vi "TEST-JSONtext-.vi"() -> ()   [LabVIEW 2019]
uses:
  3bf779cc-927d-47fd-9a8c-dc02e83297dd.vi
  <vilib>/numeric/Random Number (Range) U64.vi
  JSON-RPC/JSON-RPC.lvclass
  <vilib>/numeric/Random Number (Range) DBL.vi
  <vilib>/numeric/Random Number (Range) I64.vi
  db3575da-bffe-4b9a-a9e7-21096011e894.vi
  6d6a3817-36ec-47d6-89d3-dba7abc61dde.vi
  78cd6d8b-e620-455a-a055-8660cd06f8d0.vi
  2869ab1d-aaab-4e4d-b56e-11c366621307.vi
  740e50dd-5288-45d9-afe7-7378590220d4.vi
  7927d975-b5b9-47a3-92b0-890a8d5b504b.vi
  cbe2aa51-b106-4e40-bfc3-1c3b870f7b4b.vi
  <vilib>/ErrorRing/Error Ring.xnode
panel:
  out "spreadsheet string":string
  out "XY Graph":cluster{dbl[], dbl[]}[](graph)
  out "total":dbl format="%#_6p"
  in  "Max Response Size":i32=10000
  out "4. parse response":dbl format="%#_6p"
  out "3. create response":dbl format="%#_6p"
  out "2. parse request":dbl format="%#_6p"
  out "1. create request":dbl format="%#_6p"
  in  "method 2":string="pickFruit"
  in  "Params Type":enum16{"Array", "Cluster", "Single"}(ring)=enum."Cluster"
  in  "Num Type":enum16{"U64", "I64", "DBL"}(ring)=enum."I64"
  in  "params 2":T1={"param1"=0, "param2"=10, "param3"=10, "param2 2"=10}
  out "params":string
  out "<JSON> REQ":string
  out "error out":errorcluster
  out "id":string
  out "method":string
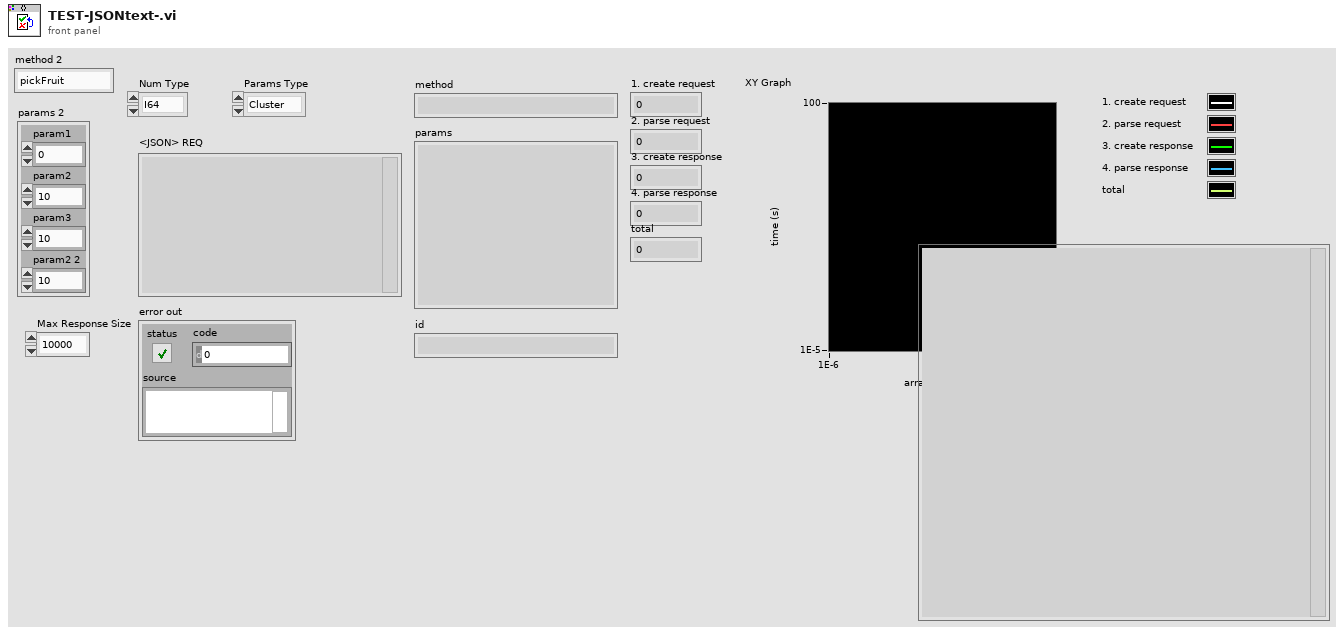
[diagram p1: front panel]
types:
  T1 = cluster{"param1":i32, "param2":i32, "param3":i32, "param2 2":i32}
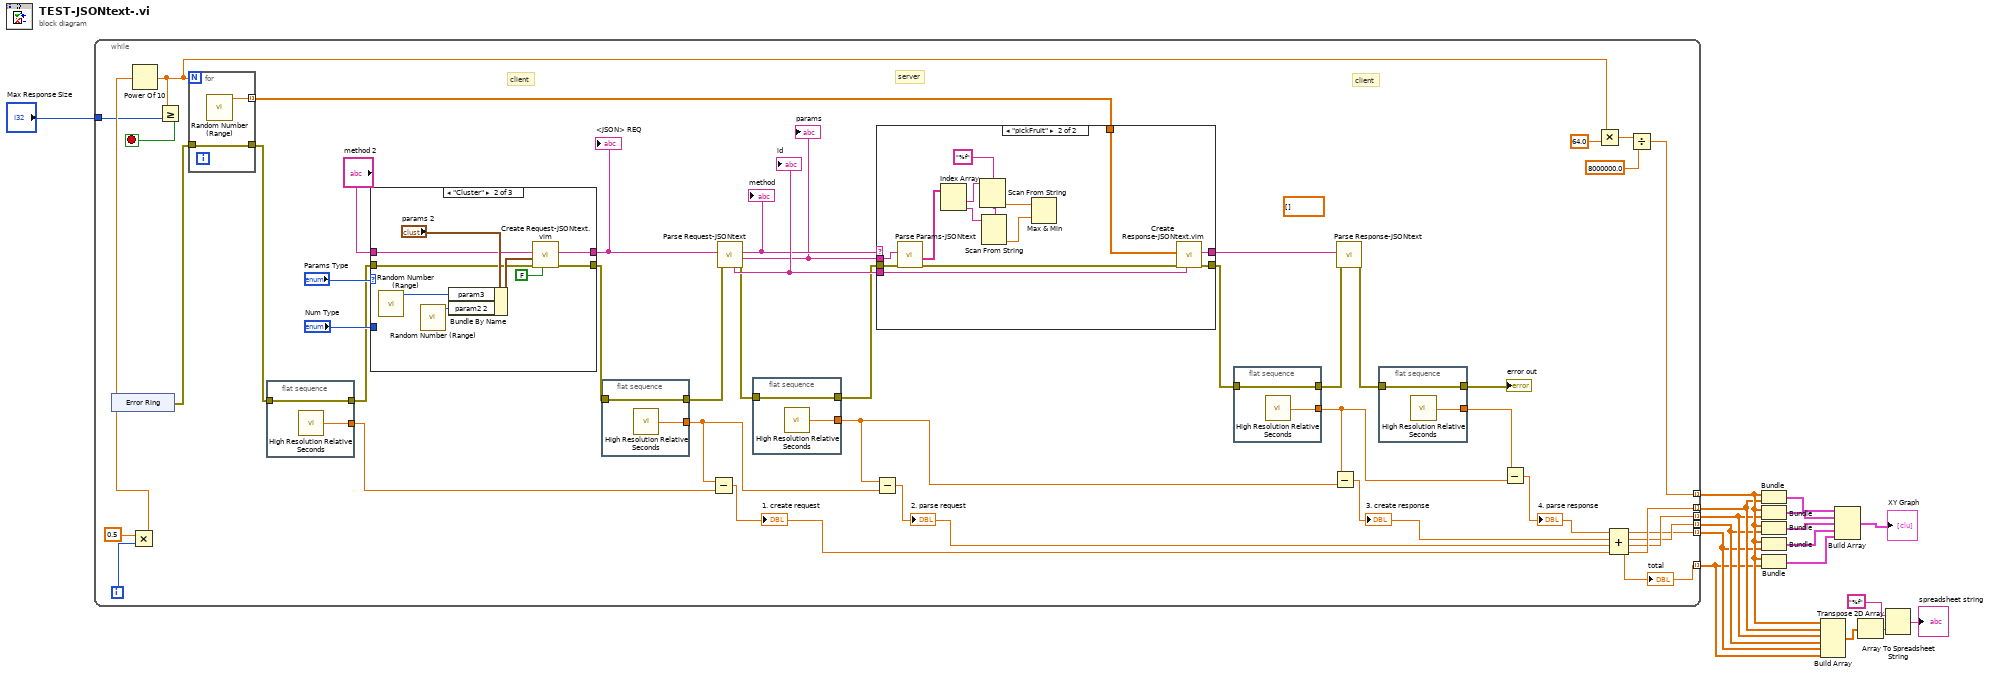
[diagram p0: block diagram]
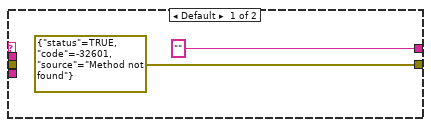
[diagram p2: hidden frame]
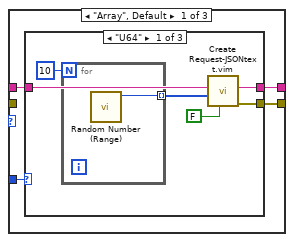
[diagram p3: hidden frame]
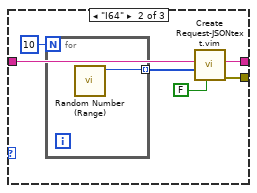
[diagram p4: hidden frame]
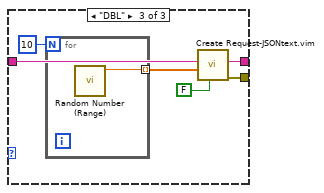
[diagram p5: hidden frame]
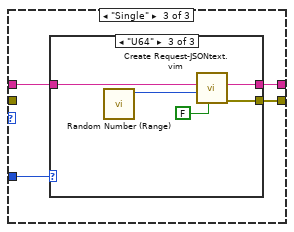
[diagram p6: hidden frame]
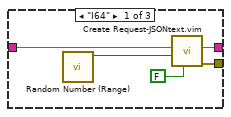
[diagram p7: hidden frame]
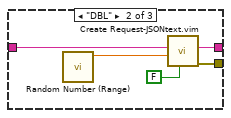
[diagram p8: hidden frame]
diagram:
  n1 = while {
    tunnel: [w32] -> w5 mode=indexing
    tunnel: [w31] -> w4 mode=indexing
    tunnel: [w30] -> w3 mode=indexing
    tunnel: [w29] -> w2 mode=indexing
    tunnel: [w28] -> w1 mode=indexing
    tunnel: [w25] -> w6 mode=indexing
    tunnel: "Max Response Size" -> [w19]
    i -> [w22]
    stop <- w18 stop-if-true
    (unwired) dbl[] []
    # "client"
    # "server"
    # "client"
    n2 = xnode "Error Ring"() -> ("error out"=w39:errorcluster)
    n3 = Multiply(x=0.5, y=w22) -> (x*y=w21:dbl)
    n4 = Power Of 10(x=w21) -> (10^x=w20:dbl)
    n5 = Greater Or Equal?(x=w20, y=w19) -> (x >= y?=w18:bool)
    n6 = for {
      N: w20 -> [_]
      tunnel: [w138] -> w33 mode=indexing
      tunnel: [w137] -> w40
      tunnel: w39 -> [w137]
      n7 = call-poly <vilib>:"Random Number (Range).vi"() -> ("number"=w138:dbl)  [unwired: 11 in]
    }
    n8 = flat-sequence {
      tunnel: w40 -> [w67]
      tunnel: [w67] -> w41
      tunnel: [w66] -> w38
      frame #0 {
        n9 = call <vilib>:"High Resolution Relative Seconds.vi"() -> ("relative seconds"=w66:dbl)
      }
    }
    n10 = case shown="\"Cluster\"" "Params Type" {
      tunnel: "Num Type" -> [w83 _ w120]
      tunnel: "method 2" -> [w84 w111 w119]
      tunnel: [w85 w110 w118] -> w49
      tunnel: [w86 w109 w117] -> w55
      tunnel: w41 -> [_ w108 _]
      frame "Array", Default {
        n11 = case shown="\"U64\"" w83 {
          tunnel: [w89 w95 w103] -> w86
          tunnel: [w90 w94 w102] -> w85
          tunnel: w84 -> [w87 w96 w101]
          frame "U64" {
            n12 = for {
              N: 10 -> [_]
              tunnel: [w93] -> w88 mode=indexing
              n13 = call-poly <vilib>:"Random Number (Range).vi"() -> ("number"=w93:u64)  [unwired: 11 in]
            }
            n14 = call "Create Request-JSONtext.vim"("notification?"=FALSE, "params"=w88, "method"=w87) -> ("error out"=w90:errorcluster, "{JSON}"=w89:string)  [unwired: 6 in, 1 out]
          }
          frame "I64" {
            n15 = for {
              N: 10 -> [_]
              tunnel: [w100] -> w97 mode=indexing
              n16 = call-poly <vilib>:"Random Number (Range).vi"() -> ("number"=w100:i64)  [unwired: 11 in]
            }
            n17 = call "Create Request-JSONtext.vim"("notification?"=FALSE, "params"=w97, "method"=w96) -> ("error out"=w94:errorcluster, "{JSON}"=w95:string)  [unwired: 6 in, 1 out]
          }
          frame "DBL" {
            n18 = for {
              N: 10 -> [_]
              tunnel: [w107] -> w104 mode=indexing
              n19 = call-poly <vilib>:"Random Number (Range).vi"() -> ("number"=w107:dbl)  [unwired: 11 in]
            }
            n20 = call "Create Request-JSONtext.vim"("notification?"=FALSE, "params"=w104, "method"=w101) -> ("error out"=w102:errorcluster, "{JSON}"=w103:string)  [unwired: 6 in, 1 out]
          }
        }
      }
      frame "Cluster" {
        n21 = call-poly <vilib>:"Random Number (Range).vi"() -> ("number"=w114:u64)  [unwired: 11 in]
        n22 = call-poly <vilib>:"Random Number (Range).vi"() -> ("number"=w115:u64)  [unwired: 11 in]
        n23 = Bundle By Name(cluster="params 2", "param3"=w114, "param2 2"=w115) -> (w112:T1)
        n24 = call "Create Request-JSONtext.vim"("notification?"=FALSE, "error in (no error)"=w108, "params"=w112, "method"=w111) -> ("error out"=w110:errorcluster, "{JSON}"=w109:string)  [unwired: 5 in, 1 out]
      }
      frame "Single" {
        n25 = case shown="\"U64\"" w120 {
          tunnel: w119 -> [w124 w129 w133]
          tunnel: [w123 w126 w131] -> w118
          tunnel: [w122 w127 w132] -> w117
          frame "I64" {
            n26 = call-poly <vilib>:"Random Number (Range).vi"() -> ("number"=w121:i64)  [unwired: 11 in]
            n27 = call "Create Request-JSONtext.vim"("notification?"=FALSE, "params"=w121, "method"=w124) -> ("error out"=w123:errorcluster, "{JSON}"=w122:string)  [unwired: 6 in, 1 out]
          }
          frame "DBL" {
            n28 = call-poly <vilib>:"Random Number (Range).vi"() -> ("number"=w128:dbl)  [unwired: 11 in]
            n29 = call "Create Request-JSONtext.vim"("notification?"=FALSE, "params"=w128, "method"=w129) -> ("error out"=w126:errorcluster, "{JSON}"=w127:string)  [unwired: 6 in, 1 out]
          }
          frame "U64" {
            n30 = call-poly <vilib>:"Random Number (Range).vi"() -> ("number"=w134:u64)  [unwired: 11 in]
            n31 = call "Create Request-JSONtext.vim"("notification?"=FALSE, "params"=w134, "method"=w133) -> ("error out"=w131:errorcluster, "{JSON}"=w132:string)  [unwired: 6 in, 1 out]
          }
        }
      }
    }
    "<JSON> REQ" <- w55
    n32 = flat-sequence {
      tunnel: w49 -> [w65]
      tunnel: [w65] -> w48
      tunnel: [w64] -> w37
      frame #0 {
        n33 = call <vilib>:"High Resolution Relative Seconds.vi"() -> ("relative seconds"=w64:dbl)
      }
    }
    n34 = Subtract(x=w37, y=w38) -> (x-y=w32:dbl)
    "1. create request" <- w32
    n35 = call "Parse Request-JSONtext.vi"("error in (no error)"=w48, "{JSON} Request"=w55) -> ("error out"=w47:errorcluster, "params"=w51:string, "method"=w52:string, "id"=w53:string)  [unwired: 6 in]
    "id" <- w53
    "params" <- w51
    "method" <- w52
    n36 = flat-sequence {
      tunnel: w47 -> [w63]
      tunnel: [w63] -> w46
      tunnel: [w62] -> w36
      frame #0 {
        n37 = call <vilib>:"High Resolution Relative Seconds.vi"() -> ("relative seconds"=w62:dbl)
      }
    }
    n38 = Subtract(x=w36, y=w37) -> (x-y=w31:dbl)
    "2. parse request" <- w31
    n39 = case shown="\"pickFruit\"" w52 {
      tunnel: w46 -> [_ w82]
      tunnel: [errorcluster {"status"=TRUE, "code"=-32601, "source"="Method not found"} ("error out") w79] -> w45
      tunnel: w51 -> [_ w81]
      tunnel: w53 -> [_ w78]
      tunnel: ["" ("{JSON}") w77] -> w50
      tunnel: w33 -> [_ w70]
      frame Default {
      }
      frame "pickFruit" {
        w75 = "%f" ("format string")
        n40 = call "Parse Params-JSONtext.vi"("error in (no error)"=w82, "JSON"=w81) -> ("error out"=w80:errorcluster, "Params"=w76:string[])  [unwired: 7 in, 1 out]
        n41 = Index Array(array=w76) -> (element #1=w73:string, element #2=w74:string)  [unwired: 2 in]
        n42 = Scan From String(format string=w75, input string=w73) -> (output 1=w72:dbl)  [unwired: 3 in, 3 out]
        n43 = Scan From String(format string=w75, input string=w74) -> (output 1=w71:dbl)  [unwired: 3 in, 3 out]
        n44 = Max & Min(x=w72, y=w71) -> ()  [unwired: 2 out]
        n45 = call "Create Response-JSONtext.vim"("id"=w78, "error in (no error)"=w80, "result"=w70) -> ("error out"=w79:errorcluster, "{JSON}"=w77:string)  [unwired: 7 in]
      }
    }
    n46 = flat-sequence {
      tunnel: w45 -> [w61]
      tunnel: [w61] -> w44
      tunnel: [w60] -> w34
      frame #0 {
        n47 = call <vilib>:"High Resolution Relative Seconds.vi"() -> ("relative seconds"=w60:dbl)
      }
    }
    n48 = Subtract(x=w34, y=w36) -> (x-y=w30:dbl)
    "3. create response" <- w30
    n49 = call "Parse Response-JSONtext.vi"("error in (no error)"=w44, "{JSON} Response"=w50) -> ("error out"=w43:errorcluster)  [unwired: 7 in, 2 out]
    n50 = flat-sequence {
      tunnel: w43 -> [w59]
      tunnel: [w59] -> w42
      tunnel: [w58] -> w35
      frame #0 {
        n51 = call <vilib>:"High Resolution Relative Seconds.vi"() -> ("relative seconds"=w58:dbl)
      }
    }
    n52 = Subtract(x=w35, y=w34) -> (x-y=w29:dbl)
    "4. parse response" <- w29
    n53 = Multiply(x=w20, y=64.0) -> (x*y=w26:dbl)
    n54 = Compound Arithmetic op=ADD(w29, w30, w31, w32) -> (w28:dbl)
    "total" <- w28
    n55 = Divide(x=w26, y=8000000.0) -> (x/y=w25:dbl)
    "error out" <- w42
  }
  n56 = Bundle(w6, w5) -> (w17:cluster{dbl[], dbl[]})  [unwired: 1 in]
  n57 = Bundle(w6, w4) -> (w16:cluster{dbl[], dbl[]})  [unwired: 1 in]
  n58 = Bundle(w6, w3) -> (w15:cluster{dbl[], dbl[]})  [unwired: 1 in]
  n59 = Bundle(w6, w2) -> (w14:cluster{dbl[], dbl[]})  [unwired: 1 in]
  n60 = Bundle(w6, w1) -> (w13:cluster{dbl[], dbl[]})  [unwired: 1 in]
  n61 = Build Array(w6, w5, w4, w3, w2, w1) -> (w10:dbl[][])
  n62 = Build Array(w17, w16, w15, w14, w13) -> (→"XY Graph":cluster{dbl[], dbl[]}[])
  n63 = Transpose 2D Array(2D array=w10) -> (transposed array=w7:dbl[][])
  n64 = Array To Spreadsheet String(array=w7, 3:"%f" ("format string")) -> (spreadsheet string=→"spreadsheet string":string)  [unwired: 1 in]
